vi "Do.vi"(8 "error in (no error)":errorcluster, 10 "Actor in":refnum<class "Actor.lvclass">, 11 "ReadData Msg":refnum<class "ReadData Msg.lvclass">) -> (0 "error out":errorcluster, 2 "Actor out":refnum<class "Actor.lvclass">)   [LabVIEW 2025, in "Task_Abstr.lvlib" / "ReadData Msg.lvclass"]
doc: "This VI delivers the message to the actor by calling the appropriate method(s) on the actor."
uses:
  ReadData Msg.lvclass
  <vilib>/ActorFramework/Actor/Actor.lvclass
  ReadData Msg.lvclass/ReadData Msg.ctl
  Task_Abstr/Task_Abstr.lvclass
  9ef47adc-f318-494c-9b8b-6df3216d6863.vi
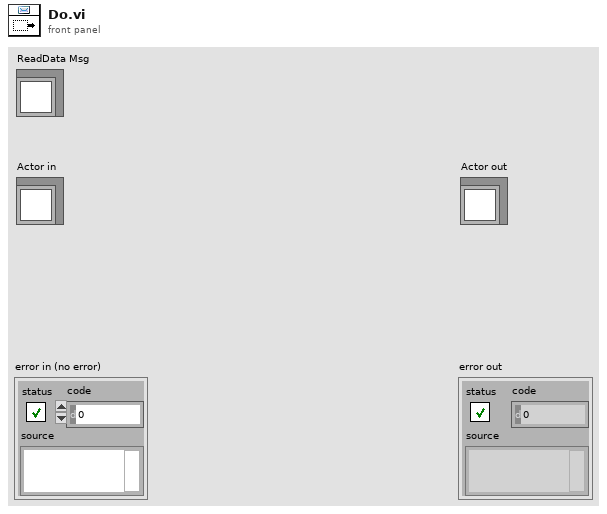
[diagram p1: front panel]
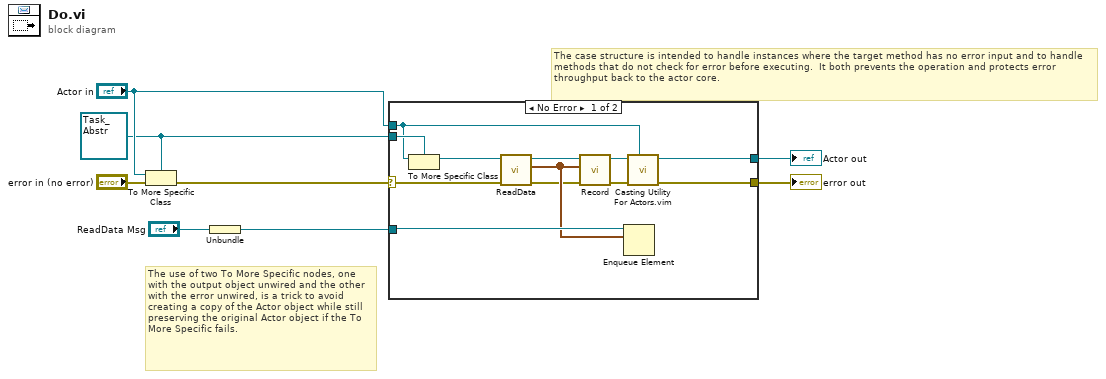
[diagram p0: block diagram]
diagram:
  w3 = refnum<class "Task_Abstr.lvclass"> refnum ("Actor in")
  # "The use of two To More Specific nodes, one with the output object unwired and the other with the error unwired, is a trick to avoid creating a copy of the Actor object while still preserving the original Actor object if the To More Specific fails."
  # "The case structure is intended to handle instances where the target method has no error input and to handle methods that do not check for error before executing.  It both prevents the operation and protects error throughput back to the actor core."
  n1 = To More Specific Class(target class=w3, reference="Actor in", error in="error in (no error)") -> (error out=w7:errorcluster)  [unwired: 1 out]
  n2 = Unbundle("ReadData Msg") -> (w1:refnum<queue>)
  n3 = case shown="No Error" w7 {
    selector: w7 -> [w20 w22]
    tunnel: [w15 w22] -> w6
    tunnel: [w16 w21] -> w5
    tunnel: "Actor in" -> [w17 w21]
    tunnel: w3 -> [w18 _]
    tunnel: w1 -> [w14 _]
    frame No Error {
      n4 = To More Specific Class(target class=w18, reference=w17) -> (specific class reference=w19:refnum<class "Task_Abstr.lvclass">)  [unwired: 1 in, 1 out]
      n5 = call-dynamic "ReadData.vi"("error in (no error)"=w20, "Task_Abstr in"=w19) -> ("error out"=w10:errorcluster, "Waveform"=w13:waveform(dbl)[], "Task_Abstr out"=w12:refnum<class "Task_Abstr.lvclass">)  [unwired: 7 in]
      n6 = call-dynamic "Record.vi"("error in (no error)"=w10, "Waveform"=w13, "Task_Abstr in"=w12) -> ("error out"=w9:errorcluster, "Task_Abstr out"=w11:refnum<class "Task_Abstr.lvclass">)  [unwired: 7 in]
      n7 = Enqueue Element(queue=w14, element=w13) -> ()  [unwired: 2 in, 3 out]
      n8 = call "Casting Utility For Actors.vim"("type"=w17, "error in (no error)"=w9, "Actor in"=w11) -> ("error out"=w15:errorcluster, "Actor out"=w16:refnum<class "Actor.lvclass">)  [unwired: 7 in]
    }
    frame Error {
      # "If type check fails, pass the original object out again."
    }
  }
  "error out" <- w6
  "Actor out" <- w5
